vi "Lift Trapazoidal Ramp.vi"(1 "Encoder":dbl, 2 "Reset":bool, 3 "Increase":dbl format="%#_13g", 4 "lower limit":dbl=0.2 format="%#_13g", 5 "Speed (-1 to 1)":dbl, 6 "Distance (inches)":dbl) -> (0 "Speed":dbl)   [LabVIEW 2014]
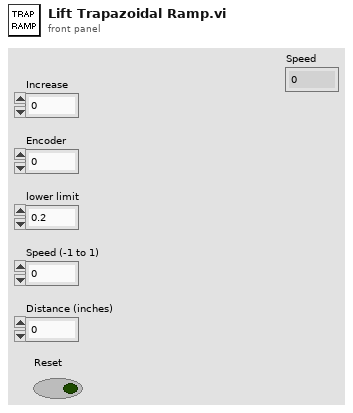
[diagram p1: front panel]
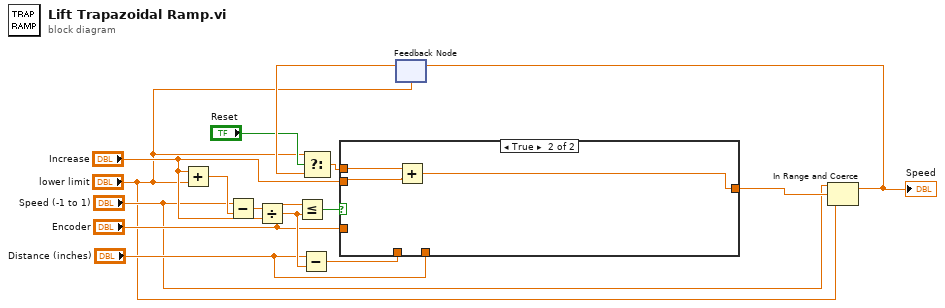
[diagram p0: block diagram]
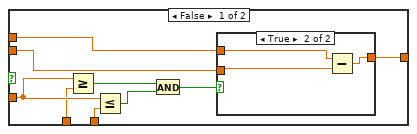
[diagram p2: hidden frame]
diagram:
  n1 = Add(x="Increase", y="lower limit") -> (x+y=w11:dbl)
  n2 = Subtract(x="Speed (-1 to 1)", y=w11) -> (x-y=w14:dbl)
  n3 = Divide(x=w14, y="Increase") -> (x/y=w13:dbl)
  n4 = Less Or Equal?(x="Encoder", y=w13) -> (x <= y?=w15:bool)
  n5 = Subtract(x="Distance (inches)", y=w13) -> (x-y=w12:dbl)
  n6 = feedback #1("lower limit") -> (w8:dbl)
  n7 = Select(t="lower limit", s="Reset", f=w8) -> (s? t:f=w7:dbl)
  n8 = case shown="True" w15 {
    tunnel: [w23 w29] -> w4
    tunnel: "Increase" -> [w24 w31]
    tunnel: w12 -> [w17 _]
    tunnel: "Encoder" -> [w18 _]
    tunnel: w7 -> [w22 w30]
    tunnel: "Distance (inches)" -> [w16 _]
    frame False {
      n9 = Greater Or Equal?(x=w18, y=w17) -> (x >= y?=w21:bool)
      n10 = Less Or Equal?(x=w18, y=w16) -> (x <= y?=w19:bool)
      n11 = And(x=w21, y=w19) -> (x .and. y?=w20:bool)
      n12 = case shown="True" w20 {
        tunnel: [w25 w28] -> w23
        tunnel: w24 -> [_ w27]
        tunnel: w22 -> [w25 w26]
        frame False {
        }
        frame True {
          n13 = Subtract(x=w26, y=w27) -> (x-y=w28:dbl)
        }
      }
    }
    frame True {
      n14 = Add(x=w30, y=w31) -> (x+y=w29:dbl)
    }
  }
  n15 = In Range and Coerce(upper limit="Speed (-1 to 1)", x=w4, lower limit="lower limit") -> (coerced(x)=w3:dbl)  [unwired: 1 out]
  "Speed" <- w3
  n16 = feedback-in #1(w3) -> ()
